vi "Get DMA Settings.vi"(8 "error in (no error)":errorcluster, 10 "DMA Channel in":T5 {"Data Type" format="%.0x"}, 11 "FPGA addon refnum in":T1 format="%.0x") -> (0 "error out":errorcluster, 2 "DMA Settings":T2={"Number of Channels"=1, "Delacing Scheme"=enum."Interleaved", "Update Rate"=1000, "dt"=1000.0, "Mode"=enum."Continuous", "Number of Samples"=0, "DMA Host Buffer"=5} {"DMA Host Buffer" items=["1 Second"=1, "2 Seconds"=2, "5 Seconds"=5, "10 Seconds"=10]; "dt" format="%#_p"; "Update Rate" items=["1 Hz"=1, "2 Hz"=2, "5 Hz"=5, "10 Hz"=10]}, 3 "FPGA addon refnum out":T1 format="%.0x")   [LabVIEW 2021, in "FPGA Addon Bitfile Reload Unit Tests.lvclass"]
uses:
  FPGA Addon Bitfile Reload Unit Tests.lvclass
  <vilib>/NI VeriStand/Custom Device API/Custom Device Item Ref.ctl
  Addon/Addon Shared/Types/DMA Information.ctl
  Addon/Addon Shared/Types/FPGA Addon Data Type.ctl
  Addon/Addon Shared/Types/DMA Settings.ctl
  Addon/Addon Shared/Types/Delacing Scheme.ctl
  Addon/Addon Shared/Types/DMA Acquisition Mode.ctl
  Addon/Addon Shared/Types/FG Action.ctl
  <vilib>/NI VeriStand/Custom Device Tools/Custom Device Utility Library/NI VeriStand - Search for Item by Name.vi
  Addon/Addon Shared/SubVIs/Constants.vi
  <vilib>/NI VeriStand/Custom Device API/NI VeriStand - Get Item Property.vi
  <vilib>/NI VeriStand/Custom Device API/Get Item Property (U32).vi
  <vilib>/NI VeriStand/Custom Device API/Get Item Property (Double).vi
  <vilib>/NI VeriStand/Custom Device API/NI VeriStand - Set Item Property.vi
  <vilib>/NI VeriStand/Custom Device API/Set Item Property (U32).vi
  <vilib>/NI VeriStand/Custom Device API/Set Item Property (Double).vi
  Addon/Addon Shared/FPGA Addon Shared.lvlib
  <vilib>/NI VeriStand/Custom Device Tools/Custom Device Utility Library/Custom Device Utility Library.lvlib
  <vilib>/NI VeriStand/Custom Device API/Custom Device API.lvlib
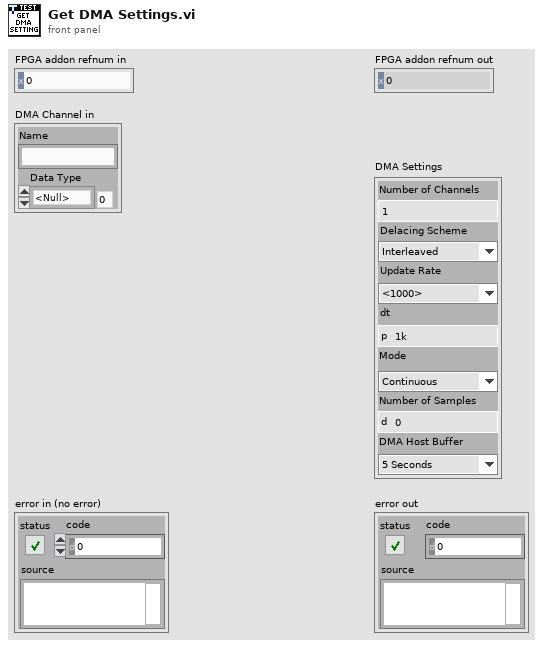
[diagram p1: front panel]
types:
  T1 = typedef "Custom Device API.lvlib/Custom Device Item Ref.ctl" = u64
  T2 = typedef "FPGA Addon Shared.lvlib/DMA Settings.ctl" = cluster{"Number of Channels":u8, "Delacing Scheme":T3, "Update Rate":u32, "dt":dbl, "Mode":T4, "Number of Samples":u32, "DMA Host Buffer":u32}
  T3 = typedef "FPGA Addon Shared.lvlib/Delacing Scheme.ctl" = enum8{"Interleaved", "Bitpacked"}
  T4 = typedef "FPGA Addon Shared.lvlib/DMA Acquisition Mode.ctl" = enum8{"Continuous", "Triggered Finite"}
  T5 = typedef "FPGA Addon Shared.lvlib/DMA Information.ctl" = cluster{"Name":string, "Data Type":T6}
  T6 = typedef "FPGA Addon Shared.lvlib/FPGA Addon Data Type.ctl" = enum8{"<Null>", "I8", "I16", "I32", "I64", "U8", "U16", "U32", "U64", "SGL", "Boolean", "Analog PWM In Settings", "Analog PWM In", "Digital PWM In Settings", "Digital PWM In", "Digital PWM Out", "Sine Out", "FXP", "FXP+/-24.5", "FXP+/-16.5", "FXP+/-32.8", "FXP+/-64.32", "FXP+/-16.7", "FXP+/-20.5", "FXP+/-27.5", "FXP+/-32.16", "FXP+16.3", "FXP+18.3", "Digital Static In", "Digital Static Out", "Digital Static In Settings", "Digital WSS Out", "Quad Encoder Settings", "Quad Encoder In", "Group"}
  T7 = typedef "FPGA Addon Shared.lvlib/FG Action.ctl" = enum8{"GET", "SET"}
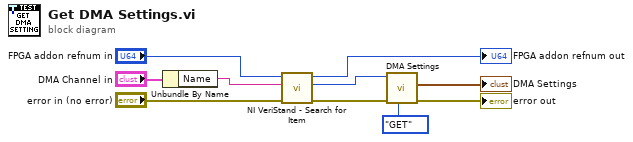
[diagram p0: block diagram]
diagram:
  n1 = Unbundle By Name("DMA Channel in") -> ("Name"=w5:string)
  n2 = call-poly <vilib>:"NI VeriStand - Search for Item.vi"("error in"="error in (no error)", "Item Name"=w5, "Section Ref in"="FPGA addon refnum in") -> ("error out"=w6:errorcluster, "Item Ref"=w7:T1, "Section Ref out"=→"FPGA addon refnum out":T1)  [unwired: 5 in, 1 out]
  n3 = call "DMA Settings.vi"("Action"=FG_Action."GET", "error in (no error)"=w6, "Item Ref"=w7) -> ("error out"=→"error out":errorcluster, "DMA Settings"=→"DMA Settings":T2)  [unwired: 6 in, 1 out]
